vi "Set Parent.vi"(8 "error in (no error)":errorcluster, 11 "LV MDI in":refnum<class "LV MDI.lvclass">) -> (0 "error out":errorcluster, 3 "LV MDI out":refnum<class "LV MDI.lvclass">)   [LabVIEW 2016, in "LV MDI.lvclass"]
uses:
  LV MDI.lvclass
  LV MDI.lvclass/LV MDI.ctl
  user32.dll
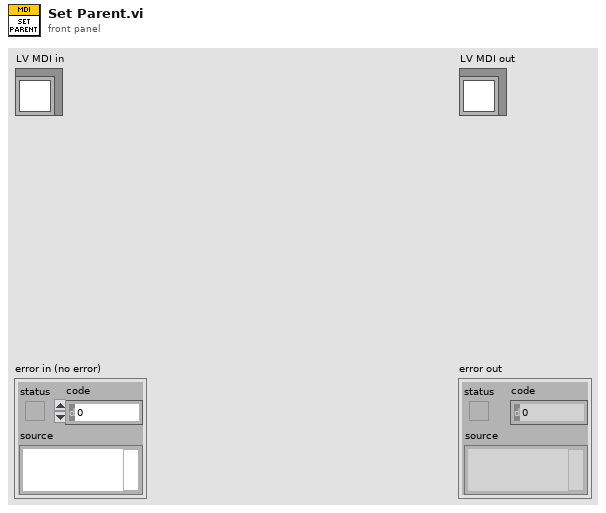
[diagram p1: front panel]
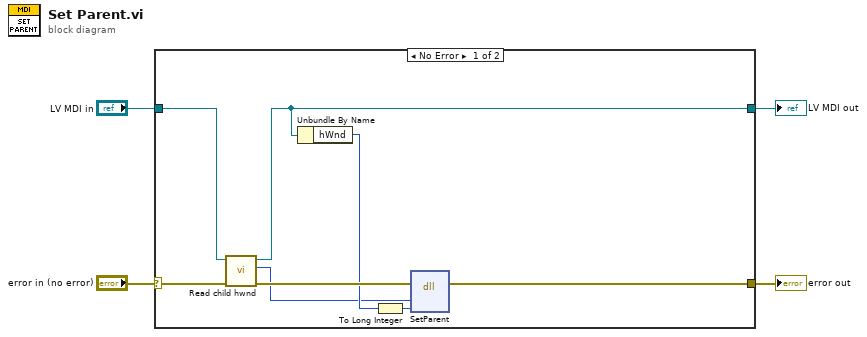
[diagram p0: block diagram]
diagram:
  n1 = case shown="No Error" "error in (no error)" {
    selector: "error in (no error)" -> [w12 w14]
    tunnel: [w7 w14] -> w3
    tunnel: [w5 w13] -> w1
    tunnel: "LV MDI in" -> [w6 w13]
    frame No Error {
      n2 = call "Read child hwnd.vi"("Error In"=w12, "LV MDI.lvclass"=w6) -> ("Error Out"=w11:errorcluster, "Child hWnd"=w8:u32, "LV MDI.lvclass"=w5:refnum<class "LV MDI.lvclass">)  [unwired: 7 in]
      n3 = Unbundle By Name(w5) -> ("hWnd"=w10:u64)
      n4 = To Long Integer(number=w10) -> (32bit integer=w9:i32)
      n5 = dll-call lib="user32.dll" fn="SetParent"(error in=w11, "Child"=w8, "NewParent"=w9) -> (error out=w7:errorcluster)  [unwired: 5 in, 1 out]
    }
    frame Error {
    }
  }
  "error out" <- w3
  "LV MDI out" <- w1
